vi "Add Subsystem Refnums.vi"(8 "error in (no error)":errorcluster, 9 "Subsystem Overview Control":refnum<vi>, 10 "Subsystem URL":refnum<k21>, 11 "Map In":variant) -> (0 "error out":errorcluster, 3 "Map Out":variant)   [LabVIEW 2024]
doc: "Adds the mapping relationship between the subsystem I/O points URL and the control refnum to the map."
uses:
  Controls/Client/Subsystem Overview.ctl
  Controls/Client/Alarm LED.ctl
  Controls/Client/Status LED.ctl
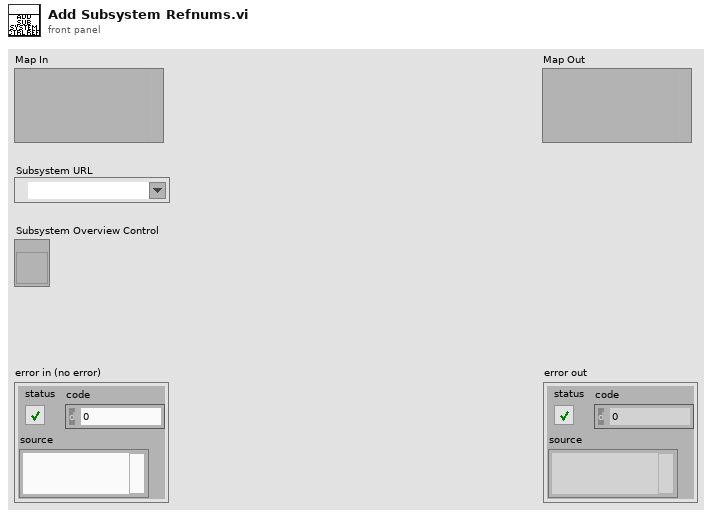
[diagram p1: front panel]
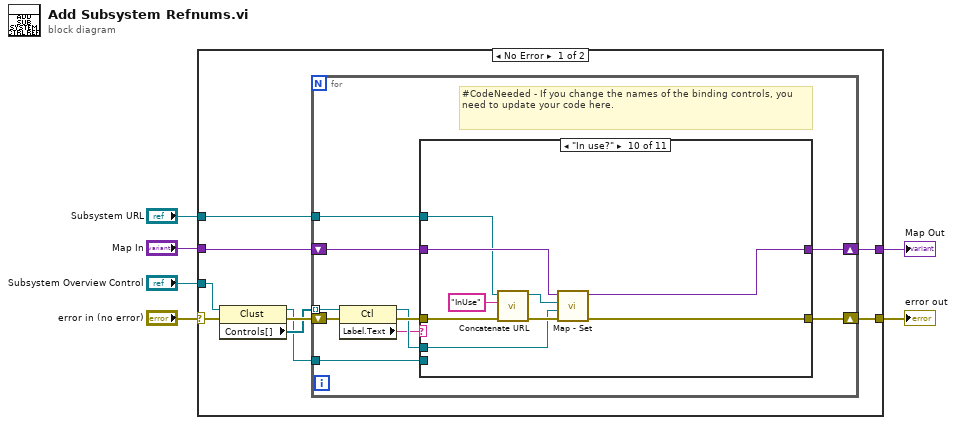
[diagram p0: block diagram]
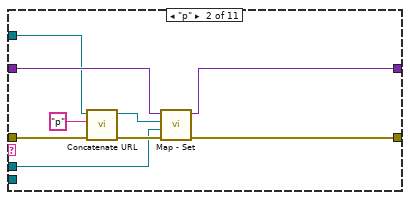
[diagram p3: hidden frame]
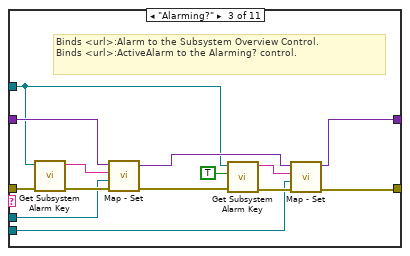
[diagram p4: hidden frame]
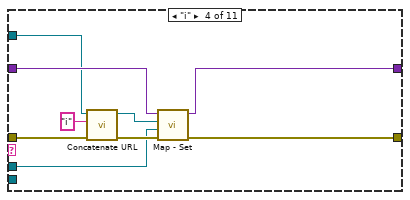
[diagram p5: hidden frame]
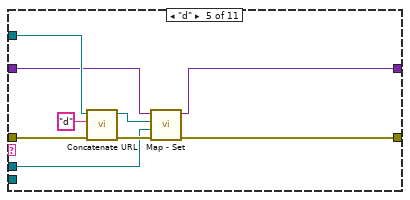
[diagram p6: hidden frame]
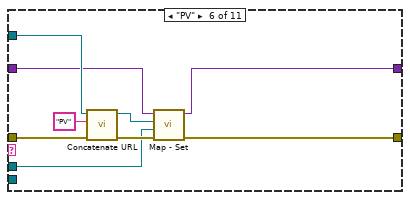
[diagram p7: hidden frame]
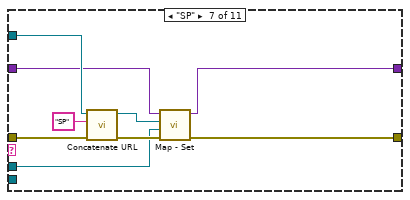
[diagram p8: hidden frame]
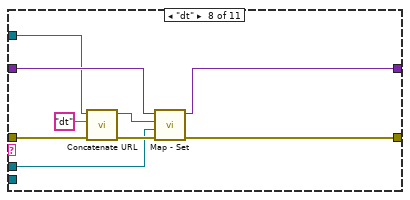
[diagram p9: hidden frame]
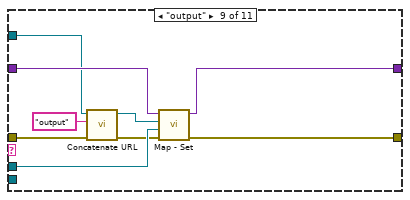
[diagram p10: hidden frame]
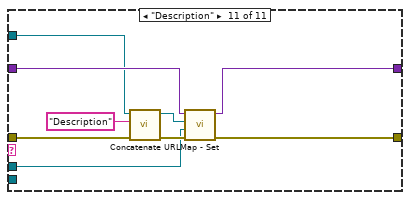
[diagram p11: hidden frame]
diagram:
  n1 = case shown="No Error" "error in (no error)" {
    selector: "error in (no error)" -> [w15 w124]
    tunnel: [w12 w124] -> w5
    tunnel: [w9 w123] -> w4
    tunnel: "Map In" -> [w10 w123]
    tunnel: "Subsystem URL" -> [w11 _]
    tunnel: "Subsystem Overview Control" -> [w14 _]
    frame No Error {
      n2 = property class="Clust"(reference=w14, error in=w15) -> (reference out=w7:refnum<vi>, error out=w13:errorcluster, "Controls[]"=w8:refnum<vi>[])
      n3 = for {
        shift-right: [w24] -> w12
        shift-left: w13 -> [w22]
        shift-right: [w23] -> w9
        shift-left: w10 -> [w25]
        tunnel: w11 -> [w18]
        tunnel: w8 -> [w17] mode=indexing
        tunnel: w7 -> [w16]
        # "#CodeNeeded - If you change the names of the binding controls, you need to update your code here."
        n4 = property class="Ctl"(reference=w17, error in=w22) -> (reference out=w20:refnum<vi>, error out=w21:errorcluster, "Label.Text"=w19:string)
        n5 = case shown="\"In use?\"" w19 {
          tunnel: w25 -> [w26 w34 w48 w53 w64 w69 w78 w90 w104 w109 w117]
          tunnel: [w27 w30 w42 w55 w62 w74 w83 w92 w103 w105 w120] -> w24
          tunnel: [w26 w29 w41 w54 w63 w75 w84 w93 w102 w106 w121] -> w23
          tunnel: w21 -> [w27 w31 w49 w57 w61 w73 w82 w91 w100 w110 w119]
          tunnel: w20 -> [_ w28 w39 w51 w60 w70 w79 w89 w101 w107 w114]
          tunnel: w18 -> [_ w33 w38 w52 w65 w71 w80 w87 w96 w108 w116]
          tunnel: w16 -> [_ _ w37 _ _ _ _ _ _ _ _]
          frame Default {
          }
          frame "p" {
            n6 = call "Concatenate URL.vi"("error in (no error)"=w31, "Child Name"="p" ("string"), "Parent URL"=w33) -> ("error out"=w35:errorcluster, "Child URL"=w36:refnum<k21>)  [unwired: 7 in]
            n7 = call "Map - Set.vi"("error in (no error)"=w35, "Value"=w28, "Key"=w36, "Map In"=w34) -> ("error out"=w30:errorcluster, "Map Out"=w29:variant)  [unwired: 5 in, 1 out]
          }
          frame "Alarming?" {
            # "Binds <url>:Alarm to the Subsystem Overview Control.\nBinds <url>:ActiveAlarm to the Alarming? control."
            n8 = call "Get Subsystem Alarm Key.vi"("error in (no error)"=w49, "Subsystem URL"=w38) -> ("error out"=w47:errorcluster, "Subsystem Alarm Key"=w50:string)  [unwired: 8 in]
            n9 = call "Map - Set.vi"("error in (no error)"=w47, "Value"=w39, "Key"=w50, "Map In"=w48) -> ("error out"=w43:errorcluster, "Map Out"=w40:variant)  [unwired: 5 in, 1 out]
            n10 = call "Get Subsystem Alarm Key.vi"("error in (no error)"=w43, "Active Alarm?"=TRUE, "Subsystem URL"=w38) -> ("error out"=w46:errorcluster, "Subsystem Alarm Key"=w45:string)  [unwired: 7 in]
            n11 = call "Map - Set.vi"("error in (no error)"=w46, "Value"=w37, "Key"=w45, "Map In"=w40) -> ("error out"=w42:errorcluster, "Map Out"=w41:variant)  [unwired: 5 in, 1 out]
          }
          frame "i" {
            n12 = call "Concatenate URL.vi"("error in (no error)"=w57, "Child Name"="i" ("string"), "Parent URL"=w52) -> ("error out"=w58:errorcluster, "Child URL"=w59:refnum<k21>)  [unwired: 7 in]
            n13 = call "Map - Set.vi"("error in (no error)"=w58, "Value"=w51, "Key"=w59, "Map In"=w53) -> ("error out"=w55:errorcluster, "Map Out"=w54:variant)  [unwired: 5 in, 1 out]
          }
          frame "d" {
            n14 = call "Concatenate URL.vi"("error in (no error)"=w61, "Child Name"="d" ("string"), "Parent URL"=w65) -> ("error out"=w67:errorcluster, "Child URL"=w68:refnum<k21>)  [unwired: 7 in]
            n15 = call "Map - Set.vi"("error in (no error)"=w67, "Value"=w60, "Key"=w68, "Map In"=w64) -> ("error out"=w62:errorcluster, "Map Out"=w63:variant)  [unwired: 5 in, 1 out]
          }
          frame "PV" {
            n16 = call "Concatenate URL.vi"("error in (no error)"=w73, "Child Name"="PV" ("string"), "Parent URL"=w71) -> ("error out"=w76:errorcluster, "Child URL"=w77:refnum<k21>)  [unwired: 7 in]
            n17 = call "Map - Set.vi"("error in (no error)"=w76, "Value"=w70, "Key"=w77, "Map In"=w69) -> ("error out"=w74:errorcluster, "Map Out"=w75:variant)  [unwired: 5 in, 1 out]
          }
          frame "SP" {
            n18 = call "Concatenate URL.vi"("error in (no error)"=w82, "Child Name"="SP" ("string"), "Parent URL"=w80) -> ("error out"=w85:errorcluster, "Child URL"=w86:refnum<k21>)  [unwired: 7 in]
            n19 = call "Map - Set.vi"("error in (no error)"=w85, "Value"=w79, "Key"=w86, "Map In"=w78) -> ("error out"=w83:errorcluster, "Map Out"=w84:variant)  [unwired: 5 in, 1 out]
          }
          frame "dt" {
            n20 = call "Concatenate URL.vi"("error in (no error)"=w91, "Child Name"="dt" ("string"), "Parent URL"=w87) -> ("error out"=w94:errorcluster, "Child URL"=w95:refnum<k21>)  [unwired: 7 in]
            n21 = call "Map - Set.vi"("error in (no error)"=w94, "Value"=w89, "Key"=w95, "Map In"=w90) -> ("error out"=w92:errorcluster, "Map Out"=w93:variant)  [unwired: 5 in, 1 out]
          }
          frame "output" {
            n22 = call "Concatenate URL.vi"("error in (no error)"=w100, "Child Name"="output" ("string"), "Parent URL"=w96) -> ("error out"=w99:errorcluster, "Child URL"=w98:refnum<k21>)  [unwired: 7 in]
            n23 = call "Map - Set.vi"("error in (no error)"=w99, "Value"=w101, "Key"=w98, "Map In"=w104) -> ("error out"=w103:errorcluster, "Map Out"=w102:variant)  [unwired: 5 in, 1 out]
          }
          frame "In use?" {
            n24 = call "Concatenate URL.vi"("error in (no error)"=w110, "Child Name"="InUse" ("string"), "Parent URL"=w108) -> ("error out"=w111:errorcluster, "Child URL"=w112:refnum<k21>)  [unwired: 7 in]
            n25 = call "Map - Set.vi"("error in (no error)"=w111, "Value"=w107, "Key"=w112, "Map In"=w109) -> ("error out"=w105:errorcluster, "Map Out"=w106:variant)  [unwired: 5 in, 1 out]
          }
          frame "Description" {
            n26 = call "Concatenate URL.vi"("error in (no error)"=w119, "Child Name"="Description" ("string"), "Parent URL"=w116) -> ("error out"=w118:errorcluster, "Child URL"=w122:refnum<k21>)  [unwired: 7 in]
            n27 = call "Map - Set.vi"("error in (no error)"=w118, "Value"=w114, "Key"=w122, "Map In"=w117) -> ("error out"=w120:errorcluster, "Map Out"=w121:variant)  [unwired: 5 in, 1 out]
          }
        }
      }
    }
    frame Error {
    }
  }
  "error out" <- w5
  "Map Out" <- w4
